vi "TimeData.vi"(0 "Action":T1(ring), 1 "Array No.":i32, 2 "Array Size / Index":i32, 3 "Data IN":u32 format="%<%H:%M:%S>t", 4 "Array IN":u32[](array[numeric]) format="%<%H:%M:%S>t") -> (5 "Data OUT":u32 format="%<%H:%M:%S>t", 6 "Array OUT":u32[](array[numeric]) format="%<%H:%M:%S>t")   [LabVIEW 2013]
doc: "Reset data arrays, or read/write array elements, or read entire\narrays.\nAction: 0 Reset arrays\n 1 Read array\n 2 Read array element\n 3 Write array element"
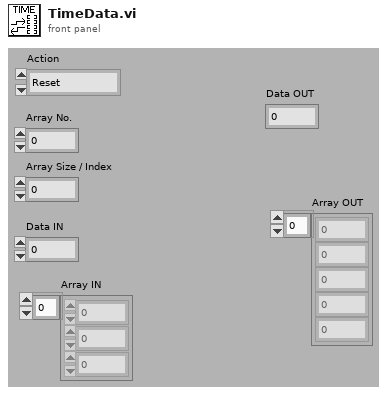
[diagram p1: front panel]
types:
  T1 = enum16{"Reset", "Read Array", "Read Element", "Write Element", "Write Array", "Add Element", "Add Array"}
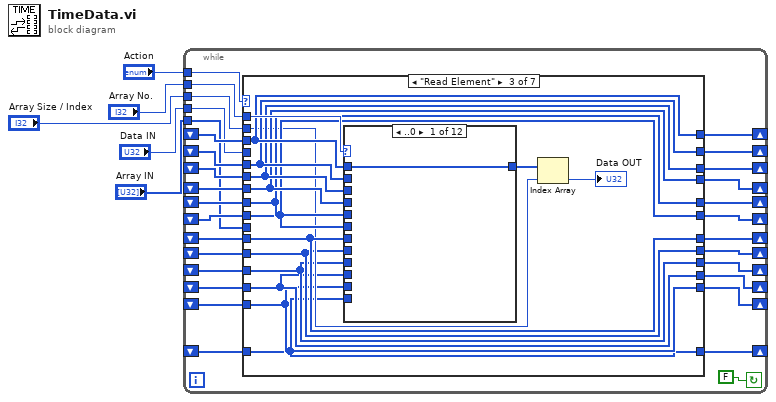
[diagram p0: block diagram]
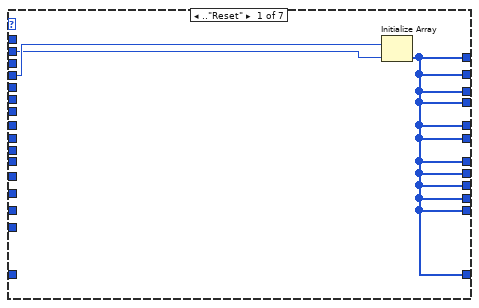
[diagram p2: hidden frame]
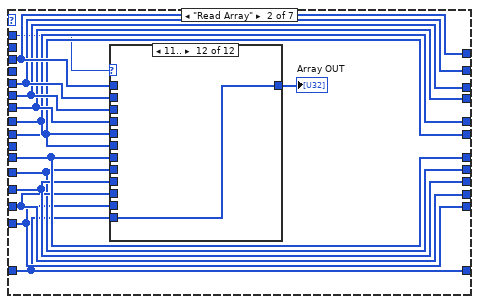
[diagram p3: hidden frame]
diagram:
  n1 = while {
    shift-left: _ -> [w15]
    shift-right: [w14] -> _
    tunnel: "Array No." -> [w16]
    shift-left: _ -> [w17]
    shift-right: [w25] -> _
    shift-left: _ -> [w18]
    shift-right: [w13] -> _
    shift-left: _ -> [w19]
    shift-right: [w26] -> _
    shift-left: _ -> [w20]
    shift-right: [w27] -> _
    shift-left: _ -> [w21]
    shift-right: [w28] -> _
    shift-left: _ -> [w22]
    shift-right: [w29] -> _
    shift-left: _ -> [w23]
    shift-right: [w30] -> _
    shift-left: _ -> [w24]
    shift-right: [w31] -> _
    tunnel: "Data IN" -> [w33]
    tunnel: "Array Size / Index" -> [w11]
    tunnel: "Action" -> [w35]
    shift-left: _ -> [w34]
    shift-right: [w32] -> _
    tunnel: "Array IN" -> [w10]
    shift-right: [w9] -> _
    shift-left: _ -> [w7]
    shift-right: [w8] -> _
    shift-left: _ -> [w6]
    stop <- FALSE continue-if-true
    n2 = case shown="\"Read Element\"" w35 {
      tunnel: [w36 w52 w79 w115 w315 w529 w714] -> w32
      tunnel: w34 -> [_ w52 w79 w119 w326 w531 w715]
      tunnel: w11 -> [w37 _ w71 w116 w324 _ _]
      tunnel: w33 -> [w38 _ _ w117 _ w530 _]
      tunnel: [w36 w51 w77 w106 w314 w527 w713] -> w31
      tunnel: [w36 w50 w76 w105 w313 w524 w712] -> w30
      tunnel: [w36 w49 w75 w104 w312 w523 w711] -> w29
      tunnel: [w36 w48 w74 w101 w311 w521 w710] -> w28
      tunnel: [w36 w47 w73 w99 w310 w520 w709] -> w27
      tunnel: [w36 w46 w72 w103 w309 w519 w708] -> w26
      tunnel: [w36 w42 w69 w97 w308 w518 w707] -> w13
      tunnel: [w36 w45 w68 w98 w307 w512 w706] -> w25
      tunnel: w24 -> [_ w51 w77 w114 w325 w528 w716]
      tunnel: w23 -> [_ w50 w76 w113 w323 w526 w717]
      tunnel: w22 -> [_ w49 w75 w112 w322 w525 w718]
      tunnel: w21 -> [_ w48 w74 w111 w321 w522 w719]
      tunnel: w20 -> [_ w47 w73 w100 w320 w517 w721]
      tunnel: w19 -> [_ w46 w72 w110 w319 w516 w722]
      tunnel: w18 -> [_ w42 w69 w109 w318 w515 w723]
      tunnel: w17 -> [_ w45 w68 w108 w317 w514 w724]
      tunnel: w16 -> [_ w44 w80 w118 w305 w532 w726]
      tunnel: w15 -> [_ w43 w67 w107 w316 w513 w725]
      tunnel: [w36 w43 w67 w102 w306 w511 w705] -> w14
      tunnel: w10 -> [_ _ _ _ w304 _ w720]
      tunnel: [w36 w41 w66 w95 w302 w507 w701] -> w9
      tunnel: [w36 w40 w65 w93 w300 w508 w702] -> w8
      tunnel: w7 -> [_ w41 w66 w96 w303 w510 w704]
      tunnel: w6 -> [_ w40 w65 w94 w301 w509 w703]
      frame .."Reset" {
        n3 = Initialize Array(w38, w37) -> (w36:u32[])
      }
      frame "Read Array" {
        n4 = case shown="11.." w44 {
          tunnel: w52 -> [w53 _ _ _ _ _ _ _ _ _ _ _]
          tunnel: [w53 w54 w55 w56 w57 w58 w59 w60 w61 w62 w63 w64] -> w39
          tunnel: w51 -> [_ w54 _ _ _ _ _ _ _ _ _ _]
          tunnel: w50 -> [_ _ w55 _ _ _ _ _ _ _ _ _]
          tunnel: w49 -> [_ _ _ w56 _ _ _ _ _ _ _ _]
          tunnel: w48 -> [_ _ _ _ w57 _ _ _ _ _ _ _]
          tunnel: w47 -> [_ _ _ _ _ w58 _ _ _ _ _ _]
          tunnel: w46 -> [_ _ _ _ _ _ w59 _ _ _ _ _]
          tunnel: w42 -> [_ _ _ _ _ _ _ w60 _ _ _ _]
          tunnel: w45 -> [_ _ _ _ _ _ _ _ w61 _ _ _]
          tunnel: w43 -> [_ _ _ _ _ _ _ _ _ w62 _ _]
          tunnel: w41 -> [_ _ _ _ _ _ _ _ _ _ w63 _]
          tunnel: w40 -> [_ _ _ _ _ _ _ _ _ _ _ w64]
          frame ..0 {
          }
          frame 1 {
          }
          frame 2 {
          }
          frame 3 {
          }
          frame 4 {
          }
          frame 5 {
          }
          frame 6 {
          }
          frame 7 {
          }
          frame 8 {
          }
          frame 9 {
          }
          frame 10 {
          }
          frame 11.. {
          }
        }
        "Array OUT" <- w39
      }
      frame "Read Element" {
        n5 = case shown="..0" w80 {
          tunnel: w79 -> [w81 _ _ _ _ _ _ _ _ _ _ _]
          tunnel: [w81 w82 w83 w84 w85 w86 w87 w88 w89 w90 w91 w92] -> w78
          tunnel: w77 -> [_ w82 _ _ _ _ _ _ _ _ _ _]
          tunnel: w76 -> [_ _ w83 _ _ _ _ _ _ _ _ _]
          tunnel: w75 -> [_ _ _ w84 _ _ _ _ _ _ _ _]
          tunnel: w74 -> [_ _ _ _ w85 _ _ _ _ _ _ _]
          tunnel: w73 -> [_ _ _ _ _ w86 _ _ _ _ _ _]
          tunnel: w72 -> [_ _ _ _ _ _ w87 _ _ _ _ _]
          tunnel: w69 -> [_ _ _ _ _ _ _ w88 _ _ _ _]
          tunnel: w68 -> [_ _ _ _ _ _ _ _ w89 _ _ _]
          tunnel: w67 -> [_ _ _ _ _ _ _ _ _ w90 _ _]
          tunnel: w66 -> [_ _ _ _ _ _ _ _ _ _ w91 _]
          tunnel: w65 -> [_ _ _ _ _ _ _ _ _ _ _ w92]
          frame ..0 {
          }
          frame 1 {
          }
          frame 2 {
          }
          frame 3 {
          }
          frame 4 {
          }
          frame 5 {
          }
          frame 6 {
          }
          frame 7 {
          }
          frame 8 {
          }
          frame 9 {
          }
          frame 10 {
          }
          frame 11.. {
          }
        }
        n6 = Index Array(array=w78, index=w71) -> (element=→"Data OUT":u32)
      }
      frame "Write Element" {
        n7 = case shown="..0" w118 {
          tunnel: w119 -> [w132 w149 w164 w179 w194 w209 w224 w239 w254 w269 w284 w299]
          tunnel: w117 -> [w134 w148 w160 w174 w188 w202 w216 w230 w245 w260 w275 w290]
          tunnel: w116 -> [w133 w147 w159 w173 w187 w201 w215 w229 w244 w257 w274 w289]
          tunnel: [w131 w149 w164 w179 w194 w209 w224 w239 w254 w269 w284 w299] -> w115
          tunnel: w114 -> [w129 w146 w163 w178 w193 w208 w223 w238 w253 w268 w283 w298]
          tunnel: w113 -> [w128 w144 w162 w177 w192 w207 w222 w237 w252 w267 w282 w297]
          tunnel: w112 -> [w127 w143 w158 w176 w191 w206 w221 w236 w251 w266 w281 w296]
          tunnel: w111 -> [w126 w142 w157 w172 w190 w205 w220 w235 w250 w265 w280 w295]
          tunnel: w110 -> [w125 w140 w155 w170 w185 w200 w218 w233 w248 w263 w278 w293]
          tunnel: w109 -> [w124 w139 w154 w169 w184 w199 w214 w232 w247 w262 w277 w292]
          tunnel: w108 -> [w123 w138 w153 w168 w183 w198 w213 w228 w246 w261 w276 w291]
          tunnel: w107 -> [w122 w137 w152 w167 w182 w197 w212 w227 w242 w259 w273 w288]
          tunnel: [w124 w139 w154 w169 w184 w199 w214 w231 w247 w262 w277 w292] -> w97
          tunnel: [w122 w137 w152 w167 w182 w197 w212 w227 w242 w258 w273 w288] -> w102
          tunnel: [w130 w141 w156 w171 w186 w203 w219 w234 w249 w264 w279 w294] -> w99
          tunnel: w100 -> [w130 w141 w156 w171 w186 w204 w219 w234 w249 w264 w279 w294]
          tunnel: [w127 w143 w158 w175 w191 w206 w221 w236 w251 w266 w281 w296] -> w104
          tunnel: [w123 w138 w153 w168 w183 w198 w213 w228 w243 w261 w276 w291] -> w98
          tunnel: [w129 w145 w163 w178 w193 w208 w223 w238 w253 w268 w283 w298] -> w106
          tunnel: [w128 w144 w161 w177 w192 w207 w222 w237 w252 w267 w282 w297] -> w105
          tunnel: [w126 w142 w157 w172 w189 w205 w220 w235 w250 w265 w280 w295] -> w101
          tunnel: [w125 w140 w155 w170 w185 w200 w217 w233 w248 w263 w278 w293] -> w103
          tunnel: w96 -> [w121 w136 w151 w166 w181 w196 w211 w226 w241 w256 w272 w287]
          tunnel: [w121 w136 w151 w166 w181 w196 w211 w226 w241 w256 w271 w287] -> w95
          tunnel: w94 -> [w120 w135 w150 w165 w180 w195 w210 w225 w240 w255 w270 w286]
          tunnel: [w120 w135 w150 w165 w180 w195 w210 w225 w240 w255 w270 w285] -> w93
          frame ..0 {
            n8 = Replace Array Subset(array=w132, new element=w134, index=w133) -> (w131:u32[])
          }
          frame 1 {
            n9 = Replace Array Subset(array=w146, new element=w148, index=w147) -> (w145:u32[])
          }
          frame 2 {
            n10 = Replace Array Subset(array=w162, new element=w160, index=w159) -> (w161:u32[])
          }
          frame 3 {
            n11 = Replace Array Subset(array=w176, new element=w174, index=w173) -> (w175:u32[])
          }
          frame 4 {
            n12 = Replace Array Subset(array=w190, new element=w188, index=w187) -> (w189:u32[])
          }
          frame 5 {
            n13 = Replace Array Subset(array=w204, new element=w202, index=w201) -> (w203:u32[])
          }
          frame 6 {
            n14 = Replace Array Subset(array=w218, new element=w216, index=w215) -> (w217:u32[])
          }
          frame 7 {
            n15 = Replace Array Subset(array=w232, new element=w230, index=w229) -> (w231:u32[])
          }
          frame 8 {
            n16 = Replace Array Subset(array=w246, new element=w245, index=w244) -> (w243:u32[])
          }
          frame 9 {
            n17 = Replace Array Subset(array=w259, new element=w260, index=w257) -> (w258:u32[])
          }
          frame 10 {
            n18 = Replace Array Subset(array=w272, new element=w275, index=w274) -> (w271:u32[])
          }
          frame 11.. {
            n19 = Replace Array Subset(array=w286, new element=w290, index=w289) -> (w285:u32[])
          }
        }
      }
      frame "Write Array" {
        n20 = case shown="11.." w305 {
          tunnel: w326 -> [w339 w356 w371 w386 w401 w416 w431 w446 w461 w476 w491 w506]
          tunnel: w304 -> [w341 w355 w367 w381 w395 w409 w423 w437 w452 w467 w482 w497]
          tunnel: w324 -> [w340 w354 w366 w380 w394 w408 w422 w436 w451 w464 w481 w496]
          tunnel: [w338 w356 w371 w386 w401 w416 w431 w446 w461 w476 w491 w506] -> w315
          tunnel: w325 -> [w336 w353 w370 w385 w400 w415 w430 w445 w460 w475 w490 w505]
          tunnel: w323 -> [w335 w351 w369 w384 w399 w414 w429 w444 w459 w474 w489 w504]
          tunnel: w322 -> [w334 w350 w365 w383 w398 w413 w428 w443 w458 w473 w488 w503]
          tunnel: w321 -> [w333 w349 w364 w379 w397 w412 w427 w442 w457 w472 w487 w502]
          tunnel: w319 -> [w332 w347 w362 w377 w392 w407 w425 w440 w455 w470 w485 w500]
          tunnel: w318 -> [w331 w346 w361 w376 w391 w406 w421 w439 w454 w469 w484 w499]
          tunnel: w317 -> [w330 w345 w360 w375 w390 w405 w420 w435 w453 w468 w483 w498]
          tunnel: w316 -> [w329 w344 w359 w374 w389 w404 w419 w434 w449 w466 w477 w495]
          tunnel: [w331 w346 w361 w376 w391 w406 w421 w438 w454 w469 w484 w499] -> w308
          tunnel: [w329 w344 w359 w374 w389 w404 w419 w434 w449 w465 w477 w495] -> w306
          tunnel: [w337 w348 w363 w378 w393 w410 w426 w441 w456 w471 w486 w501] -> w310
          tunnel: w320 -> [w337 w348 w363 w378 w393 w411 w426 w441 w456 w471 w486 w501]
          tunnel: [w334 w350 w365 w382 w398 w413 w428 w443 w458 w473 w488 w503] -> w312
          tunnel: [w330 w345 w360 w375 w390 w405 w420 w435 w450 w468 w483 w498] -> w307
          tunnel: [w336 w352 w370 w385 w400 w415 w430 w445 w460 w475 w490 w505] -> w314
          tunnel: [w335 w351 w368 w384 w399 w414 w429 w444 w459 w474 w489 w504] -> w313
          tunnel: [w333 w349 w364 w379 w396 w412 w427 w442 w457 w472 w487 w502] -> w311
          tunnel: [w332 w347 w362 w377 w392 w407 w424 w440 w455 w470 w485 w500] -> w309
          tunnel: w303 -> [w328 w343 w358 w373 w388 w403 w418 w433 w448 w463 w479 w494]
          tunnel: [w328 w343 w358 w373 w388 w403 w418 w433 w448 w463 w478 w494] -> w302
          tunnel: w301 -> [w327 w342 w357 w372 w387 w402 w417 w432 w447 w462 w480 w493]
          tunnel: [w327 w342 w357 w372 w387 w402 w417 w432 w447 w462 w480 w492] -> w300
          frame ..0 {
            n21 = Replace Array Subset(array=w339, new element=w341, index=w340) -> (w338:u32[])
          }
          frame 1 {
            n22 = Replace Array Subset(array=w353, new element=w355, index=w354) -> (w352:u32[])
          }
          frame 2 {
            n23 = Replace Array Subset(array=w369, new element=w367, index=w366) -> (w368:u32[])
          }
          frame 3 {
            n24 = Replace Array Subset(array=w383, new element=w381, index=w380) -> (w382:u32[])
          }
          frame 4 {
            n25 = Replace Array Subset(array=w397, new element=w395, index=w394) -> (w396:u32[])
          }
          frame 5 {
            n26 = Replace Array Subset(array=w411, new element=w409, index=w408) -> (w410:u32[])
          }
          frame 6 {
            n27 = Replace Array Subset(array=w425, new element=w423, index=w422) -> (w424:u32[])
          }
          frame 7 {
            n28 = Replace Array Subset(array=w439, new element=w437, index=w436) -> (w438:u32[])
          }
          frame 8 {
            n29 = Replace Array Subset(array=w453, new element=w452, index=w451) -> (w450:u32[])
          }
          frame 9 {
            n30 = Replace Array Subset(array=w466, new element=w467, index=w464) -> (w465:u32[])
          }
          frame 10 {
            n31 = Replace Array Subset(array=w479, new element=w482, index=w481) -> (w478:u32[])
          }
          frame 11.. {
            n32 = Replace Array Subset(array=w493, new element=w497, index=w496) -> (w492:u32[])
          }
        }
      }
      frame "Add Element" {
        n33 = case shown="5" w532 {
          tunnel: w531 -> [w546 w557 w571 w585 w599 w613 w627 w641 w655 w669 w685 w699]
          tunnel: w530 -> [w545 w559 w574 w586 w602 w614 w630 w644 w657 w671 w686 w700]
          tunnel: [w544 w557 w571 w585 w599 w613 w627 w641 w655 w669 w685 w699] -> w529
          tunnel: w528 -> [w543 w560 w570 w584 w598 w612 w626 w640 w654 w668 w684 w698]
          tunnel: [w543 w558 w570 w584 w598 w612 w626 w640 w654 w668 w684 w698] -> w527
          tunnel: w526 -> [w542 w556 w573 w583 w597 w611 w625 w639 w653 w667 w683 w697]
          tunnel: w525 -> [w541 w555 w563 w588 w596 w610 w624 w638 w652 w666 w682 w696]
          tunnel: [w542 w556 w572 w583 w597 w611 w625 w639 w653 w667 w683 w697] -> w524
          tunnel: [w541 w555 w563 w587 w596 w610 w624 w638 w652 w666 w682 w696] -> w523
          tunnel: w522 -> [w540 w554 w564 w582 w601 w609 w623 w637 w651 w665 w681 w695]
          tunnel: [w540 w554 w564 w582 w600 w609 w623 w637 w651 w665 w681 w695] -> w521
          tunnel: [w539 w553 w565 w581 w595 w615 w622 w636 w650 w664 w680 w694] -> w520
          tunnel: w517 -> [w539 w553 w565 w581 w595 w616 w622 w636 w650 w664 w680 w694]
          tunnel: w516 -> [w538 w552 w566 w580 w594 w608 w629 w635 w649 w663 w679 w693]
          tunnel: [w538 w552 w566 w580 w594 w608 w628 w635 w649 w663 w679 w693] -> w519
          tunnel: [w537 w551 w567 w579 w593 w607 w621 w643 w648 w662 w678 w692] -> w518
          tunnel: w515 -> [w537 w551 w567 w579 w593 w607 w621 w642 w648 w662 w678 w692]
          tunnel: w514 -> [w536 w550 w568 w578 w592 w606 w620 w634 w658 w661 w677 w691]
          tunnel: w513 -> [w535 w549 w569 w577 w591 w605 w619 w633 w647 w672 w675 w690]
          tunnel: [w536 w550 w568 w578 w592 w606 w620 w634 w656 w661 w677 w691] -> w512
          tunnel: [w535 w549 w569 w577 w591 w605 w619 w633 w647 w670 w675 w690] -> w511
          tunnel: w510 -> [w533 w548 w562 w576 w590 w604 w618 w632 w646 w660 w674 w689]
          tunnel: w509 -> [w534 w547 w561 w575 w589 w603 w617 w631 w645 w659 w676 w688]
          tunnel: [w534 w547 w561 w575 w589 w603 w617 w631 w645 w659 w676 w687] -> w508
          tunnel: [w533 w548 w562 w576 w590 w604 w618 w632 w646 w660 w673 w689] -> w507
          frame ..0 {
            n34 = Build Array (concatenate)(w546, w545) -> (w544:u32[])
          }
          frame 1 {
            n35 = Build Array (concatenate)(w560, w559) -> (w558:u32[])
          }
          frame 2 {
            n36 = Build Array (concatenate)(w573, w574) -> (w572:u32[])
          }
          frame 3 {
            n37 = Build Array (concatenate)(w588, w586) -> (w587:u32[])
          }
          frame 4 {
            n38 = Build Array (concatenate)(w601, w602) -> (w600:u32[])
          }
          frame 5 {
            n39 = Build Array (concatenate)(w616, w614) -> (w615:u32[])
          }
          frame 6 {
            n40 = Build Array (concatenate)(w629, w630) -> (w628:u32[])
          }
          frame 7 {
            n41 = Build Array (concatenate)(w642, w644) -> (w643:u32[])
          }
          frame 8 {
            n42 = Build Array (concatenate)(w658, w657) -> (w656:u32[])
          }
          frame 9 {
            n43 = Build Array (concatenate)(w672, w671) -> (w670:u32[])
          }
          frame 10 {
            n44 = Build Array (concatenate)(w674, w686) -> (w673:u32[])
          }
          frame 11.. {
            n45 = Build Array (concatenate)(w688, w700) -> (w687:u32[])
          }
        }
      }
      frame "Add Array".. {
        n46 = case shown="11.." w726 {
          tunnel: w725 -> [w729 w754 w763 w782 w794 w809 w824 w838 w849 w866 w869 w884]
          tunnel: w724 -> [w730 w753 w762 w781 w793 w808 w823 w837 w852 w863 w879 w893]
          tunnel: w723 -> [w731 w752 w761 w780 w792 w807 w822 w836 w848 w862 w878 w892]
          tunnel: w722 -> [w732 w751 w760 w779 w791 w806 w821 w828 w847 w861 w877 w891]
          tunnel: w721 -> [w733 w750 w759 w778 w790 w799 w818 w827 w846 w860 w876 w890]
          tunnel: w720 -> [w740 w747 w768 w777 w796 w810 w820 w832 w851 w865 w880 w894]
          tunnel: w719 -> [w734 w749 w758 w771 w795 w804 w817 w829 w845 w859 w875 w889]
          tunnel: w718 -> [w735 w748 w757 w776 w788 w803 w813 w830 w844 w858 w874 w888]
          tunnel: w717 -> [w736 w743 w766 w772 w787 w802 w814 w833 w843 w857 w873 w887]
          tunnel: w716 -> [w738 w744 w764 w773 w786 w801 w815 w834 w842 w856 w872 w886]
          tunnel: w715 -> [w737 w745 w765 w774 w785 w800 w816 w835 w841 w855 w871 w885]
          tunnel: [w739 w745 w765 w774 w785 w800 w816 w835 w841 w855 w871 w885] -> w714
          tunnel: [w738 w746 w764 w773 w786 w801 w815 w834 w842 w856 w872 w886] -> w713
          tunnel: [w736 w743 w767 w772 w787 w802 w814 w833 w843 w857 w873 w887] -> w712
          tunnel: [w735 w748 w757 w775 w788 w803 w813 w830 w844 w858 w874 w888] -> w711
          tunnel: [w734 w749 w758 w771 w789 w804 w817 w829 w845 w859 w875 w889] -> w710
          tunnel: [w733 w750 w759 w778 w790 w805 w818 w827 w846 w860 w876 w890] -> w709
          tunnel: [w732 w751 w760 w779 w791 w806 w819 w828 w847 w861 w877 w891] -> w708
          tunnel: [w731 w752 w761 w780 w792 w807 w822 w831 w848 w862 w878 w892] -> w707
          tunnel: [w730 w753 w762 w781 w793 w808 w823 w837 w850 w863 w879 w893] -> w706
          tunnel: [w729 w754 w763 w782 w794 w809 w824 w838 w849 w864 w869 w884] -> w705
          tunnel: w704 -> [w727 w742 w756 w770 w784 w798 w812 w826 w840 w854 w868 w883]
          tunnel: w703 -> [w728 w741 w755 w769 w783 w797 w811 w825 w839 w853 w870 w882]
          tunnel: [w728 w741 w755 w769 w783 w797 w811 w825 w839 w853 w870 w881] -> w702
          tunnel: [w727 w742 w756 w770 w784 w798 w812 w826 w840 w854 w867 w883] -> w701
          frame ..0 {
            n47 = Build Array (concatenate)(w737, w740) -> (w739:u32[])
          }
          frame 1 {
            n48 = Build Array (concatenate)(w744, w747) -> (w746:u32[])
          }
          frame 2 {
            n49 = Build Array (concatenate)(w766, w768) -> (w767:u32[])
          }
          frame 3 {
            n50 = Build Array (concatenate)(w776, w777) -> (w775:u32[])
          }
          frame 4 {
            n51 = Build Array (concatenate)(w795, w796) -> (w789:u32[])
          }
          frame 5 {
            n52 = Build Array (concatenate)(w799, w810) -> (w805:u32[])
          }
          frame 6 {
            n53 = Build Array (concatenate)(w821, w820) -> (w819:u32[])
          }
          frame 7 {
            n54 = Build Array (concatenate)(w836, w832) -> (w831:u32[])
          }
          frame 8 {
            n55 = Build Array (concatenate)(w852, w851) -> (w850:u32[])
          }
          frame 9 {
            n56 = Build Array (concatenate)(w866, w865) -> (w864:u32[])
          }
          frame 10 {
            n57 = Build Array (concatenate)(w868, w880) -> (w867:u32[])
          }
          frame 11.. {
            n58 = Build Array (concatenate)(w882, w894) -> (w881:u32[])
          }
        }
      }
    }
  }
